vi "Read F and E Results.vi"(8 "error in (no error)":errorcluster, 11 "Analyze Results Fluence and Energy in":refnum<class "Analyze Results Fluence and Energy.lvclass">) -> (0 "error out":errorcluster, 1 "Energy":refnum<class "Analyze Results Energy.lvclass">, 2 "Fluence":refnum<class "Analyze Results Fluence.lvclass">, 3 "Analyze Results Fluence and Energy out":refnum<class "Analyze Results Fluence and Energy.lvclass">)   [LabVIEW 2014, in "Analyze Results Fluence and Energy.lvclass"]
uses:
  Analyze Results Fluence and Energy.lvclass
  Results Energy/Analyze Results Energy.lvclass
  Results Fluence/Analyze Results Fluence.lvclass
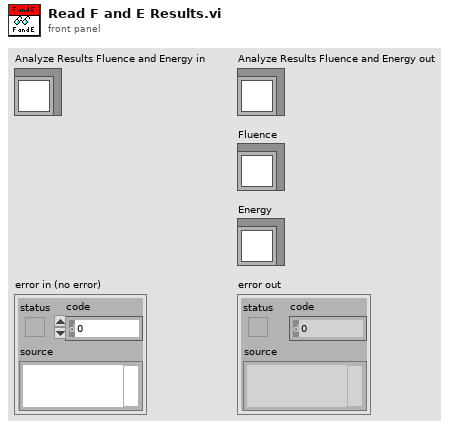
[diagram p1: front panel]
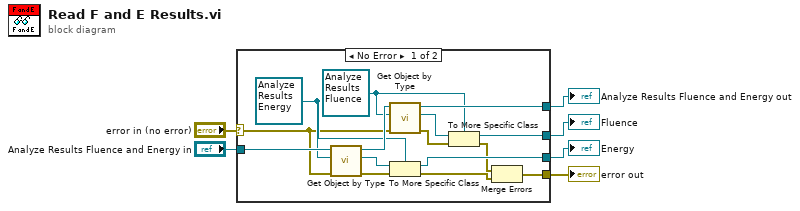
[diagram p0: block diagram]
diagram:
  n1 = case shown="No Error" "error in (no error)" {
    selector: "error in (no error)" -> [w14 w23]
    tunnel: [w7 w23] -> w5
    tunnel: [w19 w22] -> w3
    tunnel: "Analyze Results Fluence and Energy in" -> [w21 w22]
    tunnel: [w16 _] -> w2
    tunnel: [w10 _] -> w1
    frame No Error {
      w13 = refnum<class "Analyze Results Fluence.lvclass"> refnum ("Analyze Results Fluence.lvclass")
      w18 = refnum<class "Analyze Results Energy.lvclass"> refnum ("Analyze Results Energy.lvclass")
      n2 = call-dynamic "Get Object by Type.vi"("error in (no error)"=w14, "Type"=w18, "Analyze Compound Results Base in"=w21) -> ("error out"=w15:errorcluster, "Result Obj"=w17:refnum<class "Analyze Results Base.lvclass">, "Analyze Compound Results Base out"=w20:refnum<class "Analyze Results Fluence and Energy.lvclass">)  [unwired: 5 in, 1 out]
      n3 = call-dynamic "Get Object by Type.vi"("error in (no error)"=w14, "Type"=w13, "Analyze Compound Results Base in"=w20) -> ("error out"=w11:errorcluster, "Result Obj"=w12:refnum<class "Analyze Results Base.lvclass">, "Analyze Compound Results Base out"=w19:refnum<class "Analyze Results Fluence and Energy.lvclass">)  [unwired: 5 in, 1 out]
      n4 = To More Specific Class(target class=w18, reference=w17, error in=w15) -> (specific class reference=w16:refnum<class "Analyze Results Energy.lvclass">, error out=w8:errorcluster)
      n5 = To More Specific Class(target class=w13, reference=w12, error in=w11) -> (specific class reference=w10:refnum<class "Analyze Results Fluence.lvclass">, error out=w9:errorcluster)
      n6 = Merge Errors(w9, w8) -> (w7:errorcluster)
    }
    frame Error {
    }
  }
  "error out" <- w5
  "Analyze Results Fluence and Energy out" <- w3
  "Energy" <- w2
  "Fluence" <- w1
